vi "Guess-Number.vi"() -> ()   [LabVIEW 2014]
panel:
  in  "stop":bool
  out "Answer":i32
  out "Boolean":bool
  in  "You guess":dbl
  # "The answer can be invisible."
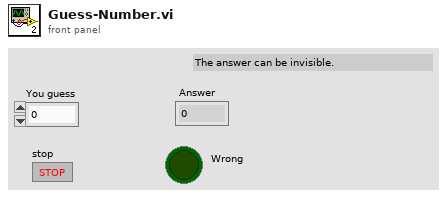
[diagram p1: front panel]
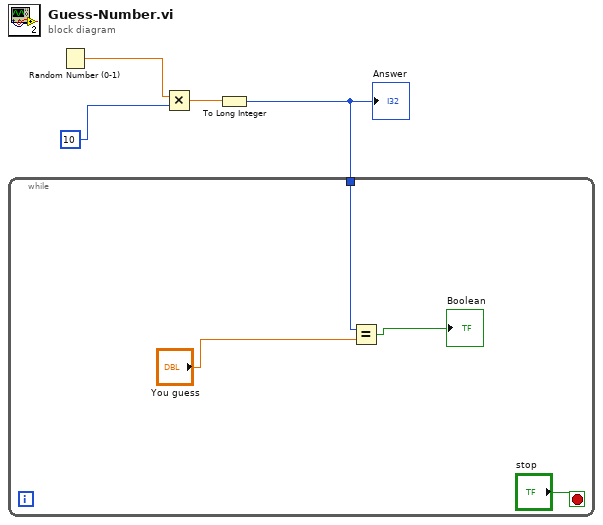
[diagram p0: block diagram]
diagram:
  n1 = Random Number (0-1)() -> (number: 0 to 1=w2:dbl)
  n2 = Multiply(x=w2, y=10) -> (x*y=w4:dbl)
  n3 = To Long Integer(number=w4) -> (32bit integer=w1:i32)
  "Answer" <- w1
  n4 = while {
    tunnel: w1 -> [w5]
    stop <- "stop" stop-if-true
    n5 = Equal?(x=w5, y="You guess") -> (x = y?=→"Boolean":bool)
  }
